vi "Send Normal or Emergency Stop.vi"(8 "error in (no error)":errorcluster, 10 "final error code":i32, 11 "Message Enqueuer":refnum<class "Message Enqueuer.lvclass">) -> (0 "error out":errorcluster)   [LabVIEW 2020, in "Actor Framework.lvlib" / "Stop Msg.lvclass"]
doc: "<p>(<strong>Filename</strong>: <span class=\"dnl\">Actor Framework.lvlib:Stop Msg.lvclass:Send Normal or Emergency Stop.vi</span>)</p>\n\n<p>Sends a Stop message to an actor. The priority of this message is determined by the value of the <strong>final error code</strong> input. If this input is <span class=\"Monospace\">0</span>, this VI sends the message with normal priority; otherwise, it sends the message with critical priority.</p>"
uses:
  Stop Msg.lvclass
  Message Enqueuer/Message Enqueuer.lvclass
  Stop Msg.lvclass/Stop Msg.ctl
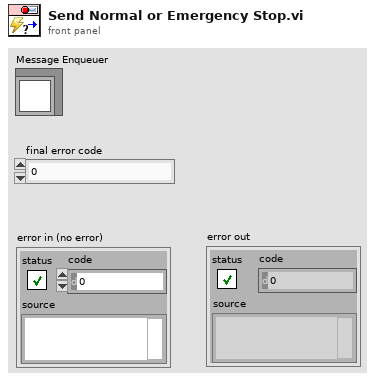
[diagram p1: front panel]
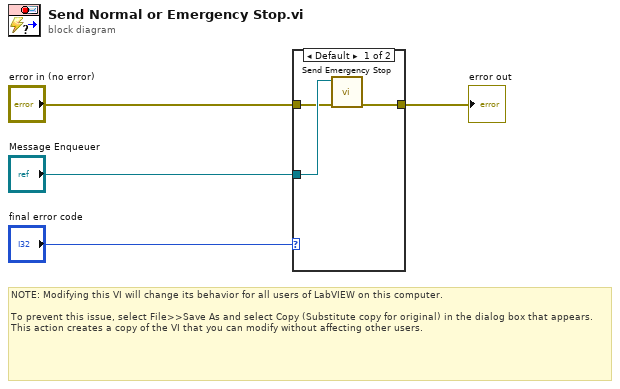
[diagram p0: block diagram]
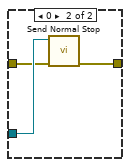
[diagram p2: hidden frame]
diagram:
  # "NOTE: Modifying this VI will change its behavior for all users of LabVIEW on this computer.\n\nTo prevent this issue, select File>>Save As and select Copy (Substitute copy for original) in the dialog box that appears. This action creates a copy of the VI that you can modify without affecting other users."
  n1 = case shown="Default" "final error code" {
    tunnel: "Message Enqueuer" -> [w7 w10]
    tunnel: "error in (no error)" -> [w6 w9]
    tunnel: [w5 w8] -> w1
    frame Default {
      n2 = call "Send Emergency Stop.vi"("error in (no error)"=w6, "Message Enqueuer"=w7) -> ("error out"=w5:errorcluster)  [unwired: 9 in]
    }
    frame 0 {
      n3 = call "Send Normal Stop.vi"("error in (no error)"=w9, "Message Enqueuer"=w10) -> ("error out"=w8:errorcluster)  [unwired: 9 in]
    }
  }
  "error out" <- w1
